vi "HTTP POST.vi"(6 "request specific headers":T1[](array[typedef]), 8 "error in (no error)":errorcluster, 9 "Request body":string, 10 "Path":string, 11 "REST Client in":refnum<class "REST Client.lvclass">) -> (0 "error out":errorcluster, 1 "Response body":string, 2 "Response headers":string, 3 "REST Client out":refnum<class "REST Client.lvclass">, 4 "Status String":string, 5 "Status Code":u16)   [LabVIEW 2013, in "REST Client.lvclass"]
uses:
  REST Client.lvclass
  HTTP Header.ctl
  HTTP Methods.ctl
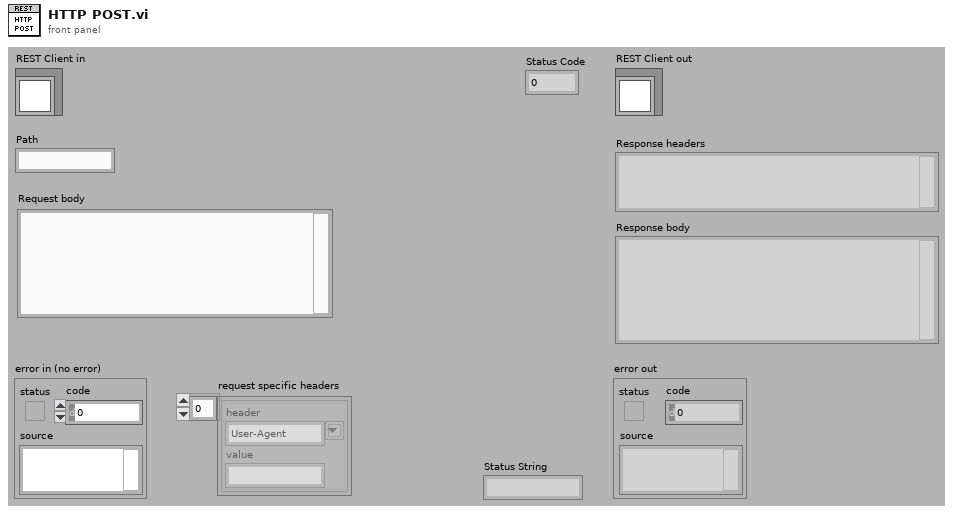
[diagram p1: front panel]
types:
  T1 = typedef "REST Client.lvclass/HTTP Header.ctl" = cluster{"header":string, "value":string}
  T2 = typedef "REST Client.lvclass/HTTP Methods.ctl" = enum16{"GET", "HEAD", "POST", "PUT", "DELETE"}
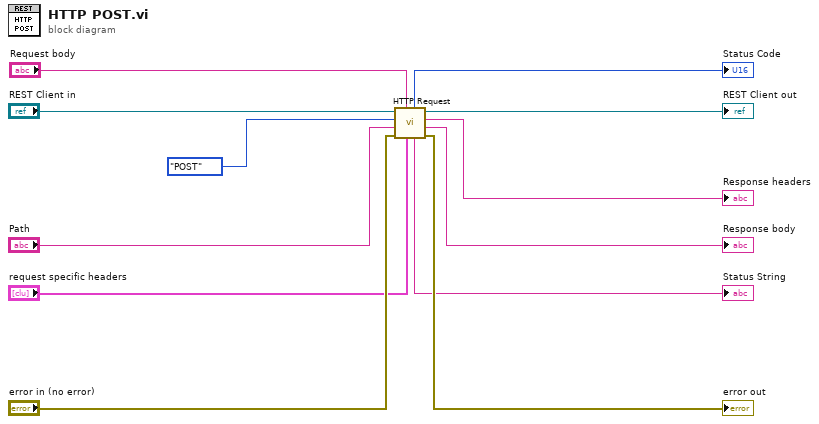
[diagram p0: block diagram]
diagram:
  n1 = call-dynamic "HTTP Request.vi"("request specific headers"="request specific headers", "Request body"="Request body", "error in (no error)"="error in (no error)", "Path"="Path", "Method"=HTTP_Methods."POST", "REST Client in"="REST Client in") -> ("error out"=→"error out":errorcluster, "Response body"=→"Response body":string, "Response headers"=→"Response headers":string, "REST Client out"=→"REST Client out":refnum<class "REST Client.lvclass">, "Status String"=→"Status String":string, "Status Code"=→"Status Code":u16)
